vi "Playbook_Init.vi"(0 "object in":refnum<class "Playbook.lvclass">, 5 "error in (no error)":errorcluster) -> (14 "object out":refnum<class "Playbook.lvclass">, 19 "error out":errorcluster)   [LabVIEW 2020, in "Playbook.lvclass"]
uses:
  Playbook.lvclass
  Play_class/Play.lvclass
  Playbook.lvclass/Playbook.ctl
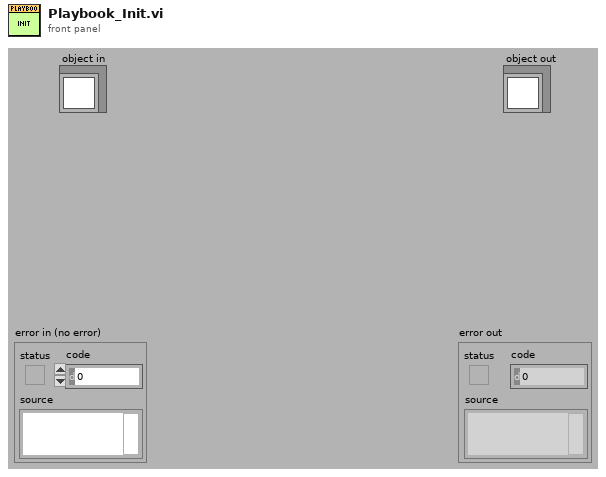
[diagram p1: front panel]
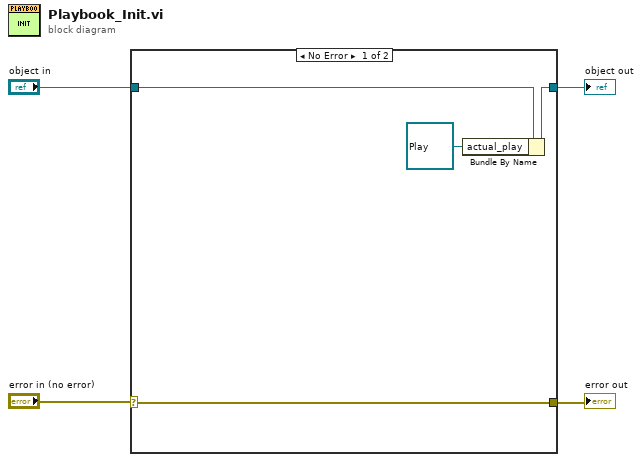
[diagram p0: block diagram]
diagram:
  n1 = case shown="No Error" "error in (no error)" {
    selector: "error in (no error)" -> [w6 w9]
    tunnel: "object in" -> [w8 w10]
    tunnel: [w7 w10] -> w3
    tunnel: [w6 w9] -> w1
    frame No Error {
      n2 = Bundle By Name(cluster=w8, "actual_play"=refnum<class "Play.lvclass"> refnum) -> (w7:refnum<class "Playbook.lvclass">)
    }
    frame Error {
    }
  }
  "object out" <- w3
  "error out" <- w1
